vi "Dataset_Reader(AutoEncoder).vi"(11 "Train dataset path":path=path "D:/working/Anomaly Detection/Train") -> (0 "error out":errorcluster, 3 "Dataset":T1)   [LabVIEW 2020]
uses:
  <vilib>/Ngene/DeepLTK/Toolkit/NN_Data/API/DataSet_Types/NN_DataSet(In1D_Out1D).ctl
  <vilib>/Ngene/DeepLTK/Toolkit/NN_Data/API/DataRef_Types/NN_Data_ref(2D_SGL).ctl
  <vilib>/Ngene/DeepLTK/Toolkit/NN_Data/API/DataRef_Types/NN_Data_ref(1D_I32).ctl
  <vilib>/Utility/file.llb/Read Delimited Spreadsheet (DBL).vi
  <vilib>/Ngene/DeepLTK/Toolkit/Deep_Learning_Toolkit_by_Ngene.lvlib
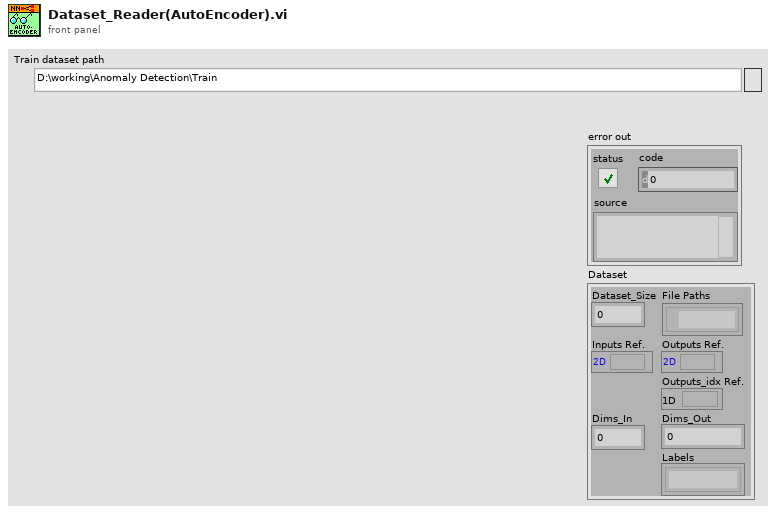
[diagram p1: front panel]
types:
  T1 = typedef "Deep_Learning_Toolkit_by_Ngene.lvlib/NN_DataSet(In1D_Out1D).ctl" = cluster{"Inputs Ref.":T2, "Outputs Ref.":T2, "Dims_In":i32, "Dataset_Size":i32, "Outputs_idx Ref.":T3, "Dims_Out":i32, "Labels":string[], "File Paths":path[]}
  T2 = typedef "Deep_Learning_Toolkit_by_Ngene.lvlib/NN_Data_ref(2D_SGL).ctl" = refnum<data-value>
  T3 = typedef "Deep_Learning_Toolkit_by_Ngene.lvlib/NN_Data_ref(1D_I32).ctl" = refnum<data-value>
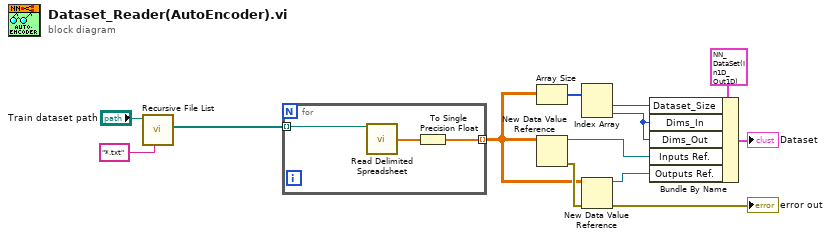
[diagram p0: block diagram]
diagram:
  n1 = call <vilib>:"Recursive File List.vi"("pattern"="*.txt", "Folder Path"="Train dataset path") -> ("All Files in Dir"=w5:path[])  [unwired: 5 in, 4 out]
  n2 = for {
    tunnel: w5 -> [w16] mode=indexing
    tunnel: [w14] -> w4 mode=indexing
    n3 = call-poly <vilib>:"Read Delimited Spreadsheet.vi"("file path (dialog if empty)"=w16) -> ("first row"=w15:dbl[])  [unwired: 9 in, 5 out]
    n4 = To Single Precision Float(number=w15) -> (single precision float=w14:sgl[])
  }
  n5 = Array Size(array=w4) -> (size(s)=w11:i32[])
  n6 = New Data Value Reference(data value=w4) -> (data value reference=w13:refnum<data-value>, error out=w10:errorcluster)  [unwired: 1 in]
  n7 = Index Array(array=w11) -> (element #1=w9:i32, element #2=w8:i32)  [unwired: 2 in]
  n8 = New Data Value Reference(data value=w4, error in=w10) -> (data value reference=w12:refnum<data-value>, error out=→"error out":errorcluster)
  n9 = Bundle By Name(cluster=T1 {"Inputs Ref."=refnum, "Outputs Ref."=refnum, "Dims_In"=0, "Dataset_Size"=0, "Outputs_idx Ref."=refnum, "Dims_Out"=0, "Labels"=[], "File Paths"=[]} ("Dataset(In1D_Out1D)"), "Dataset_Size"=w9, "Dims_In"=w8, "Dims_Out"=w8, "Inputs Ref."=w13, "Outputs Ref."=w12) -> (→"Dataset":T1)
